vi "all-signals-expressvi-to-TDMS.vi"() -> ()   [LabVIEW 2018]
panel:
  in  "Dateiname":string="test.tdms"
  in  "Dateipfad":path=path "C:/Users/lauri/OneDrive/Dokumente/Uni/HTW/Diplomarbeit/Versuchsstand neu/labview/messungen"
  in  "Stop Measurement (F)":bool caption="Messung stoppen, Counter schreiben (F)"
  in  "Clear Charts":bool
  in  "Messzeit in ms":u32=100 min=10 max=1000 step=10
  out "Bremsmoment":waveform(dbl)(graph)
  out "Strom, Spannung, elektrische Leistung":dynamicdata(graph)
  out "Counter/Messzeit":waveform(dbl)(graph)
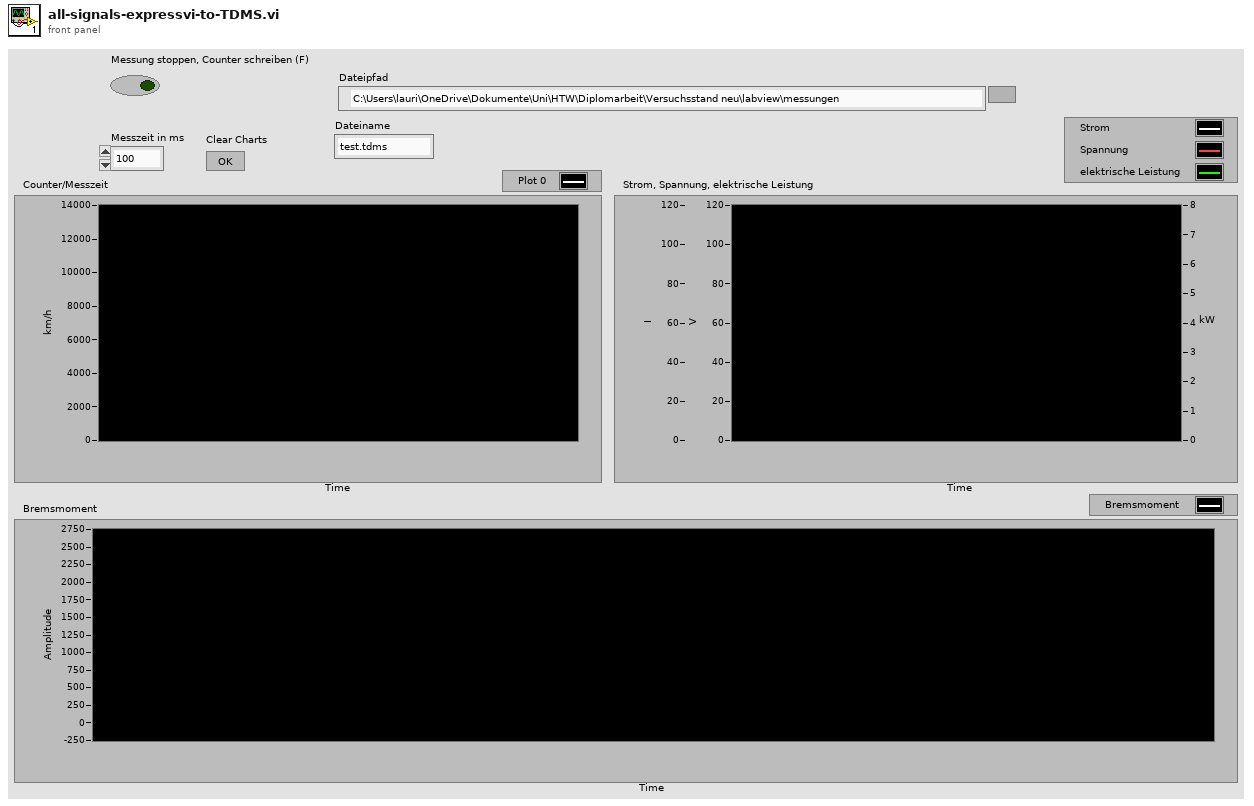
[diagram p1: front panel]
types:
  T1 = enum16{"open", "open or create", "create or replace", "create", "open (read-only)"}
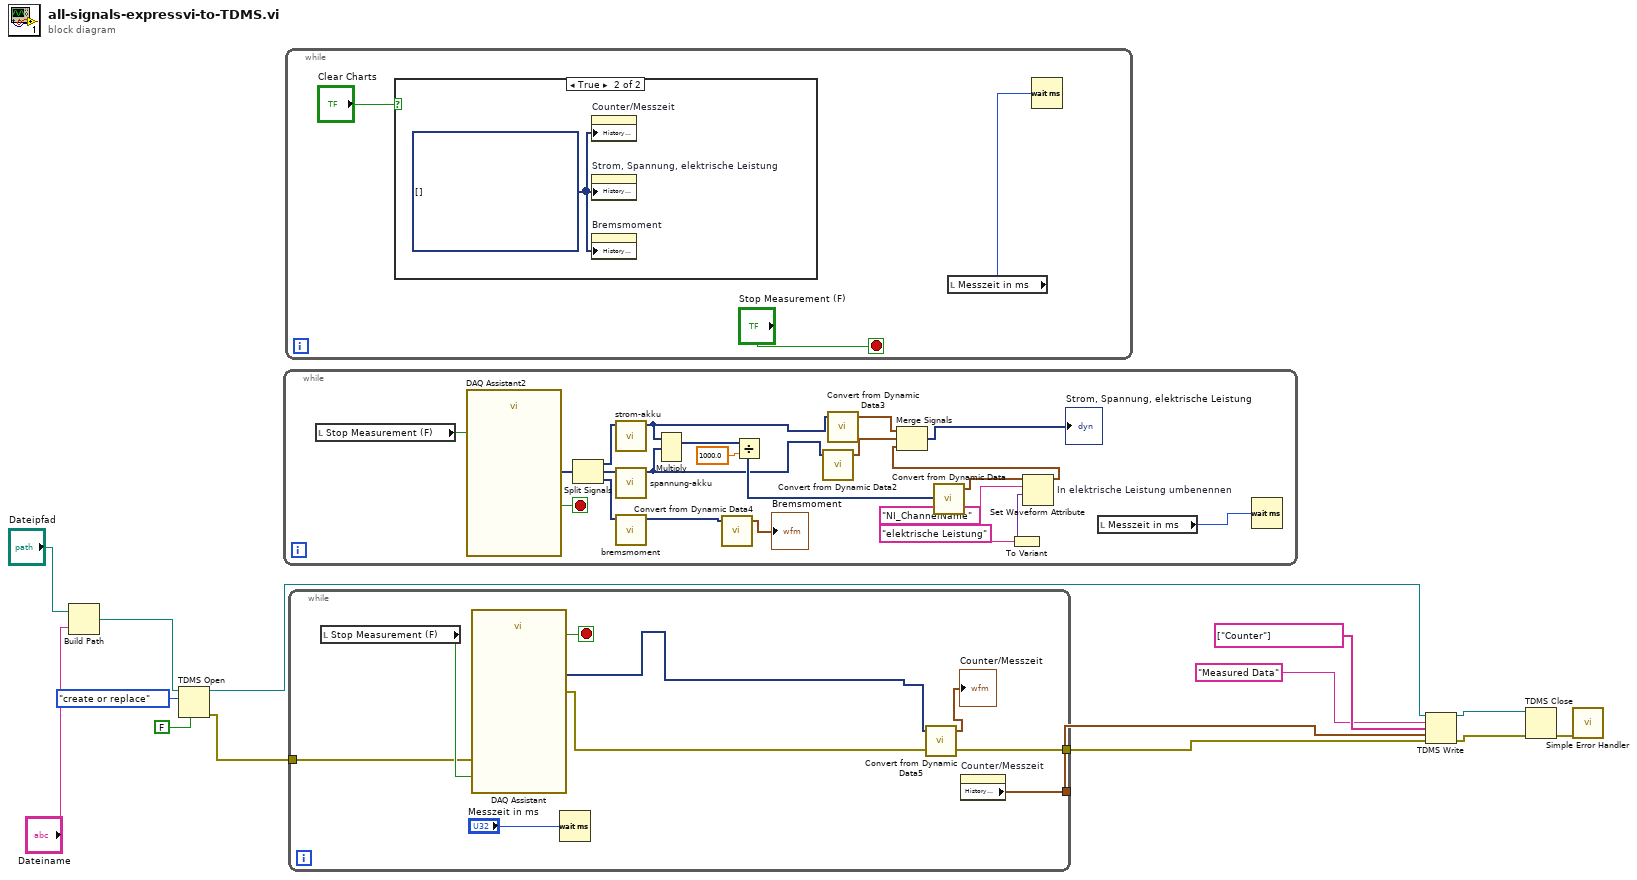
[diagram p0: block diagram]
diagram:
  n1 = Build Path(base path="Dateipfad", name or relative path="Dateiname") -> (appended path=w6:path)
  n2 = TDMS Open(6:FALSE ("disable buffering? (T)"), 10:T1."create or replace" ("operation (0:open)"), 11:w6) -> (0:w11:errorcluster, 3:w8:refnum<k34>)  [unwired: 4 in]
  n3 = while {
    stop <- w32 stop-if-true
    n4 = local read "Stop Measurement (F)"() -> (w29:bool)
    n5 = call "DAQ Assistant2"("stop (F)"=w29) -> ("data"=w33:dynamicdata, "stopped"=w32:bool)  [unwired: 15 in, 2 out]
    n6 = Split Signals(w33) -> (w36:dynamicdata, w35:dynamicdata, w34:dynamicdata)  [unwired: 3 in]
    n7 = call "strom-akku.vi"("Dynamic Data"=w36) -> ("Filtered Signal"=w20:dynamicdata)  [unwired: 10 in]
    n8 = call "spannung-akku.vi"("Dynamic Data in"=w35) -> ("Dynamic Data out"=w22:dynamicdata)  [unwired: 10 in]
    n9 = call "bremsmoment.vi"("Dynamic Data in"=w34) -> ("Dynamic Data out"=w18:dynamicdata)  [unwired: 10 in]
    n10 = Multiply(1:w22, 2:w20) -> (0:w30:dynamicdata)  [unwired: 1 in, 1 out]
    n11 = call "Convert from Dynamic Data4"("Dynamic Data Type"=w18) -> ("Waveform"=→"Bremsmoment":waveform(dbl))  [unwired: 3 in]
    n12 = Divide(x=w30, y=1000.0) -> (x/y=w28:dynamicdata)
    n13 = call "Convert from Dynamic Data2"("Dynamic Data Type"=w22) -> ("Waveform"=w21:waveform(dbl))  [unwired: 3 in]
    n14 = call "Convert from Dynamic Data3"("Dynamic Data Type"=w20) -> ("Waveform"=w19:waveform(dbl))  [unwired: 3 in]
    n15 = call "Convert from Dynamic Data"("Dynamic Data Type"=w28) -> ("Waveform"=w24:waveform(dbl))  [unwired: 3 in]
    n16 = To Variant(anything="elektrische Leistung") -> (Variant=w27:variant)
    n17 = Set Waveform Attribute "In elektrische Leistung umbenennen"(5:w27, 6:"NI_ChannelName" ("name"), 7:w24) -> (3:w23:waveform(dbl))  [unwired: 1 in, 2 out]
    n18 = Merge Signals "Merge Signals"(w19, w21, w23) -> (→"Strom, Spannung, elektrische Leistung":dynamicdata)
    n19 = local read "Messzeit in ms"() -> (w15:u32)
    n20 = Wait (ms)(milliseconds to wait=w15) -> ()  [unwired: 1 out]
  }
  n21 = while {
    stop <- "Stop Measurement (F)" stop-if-true
    n22 = case shown="True" "Clear Charts" {
      frame False {
      }
      frame True {
        w40 = dynamicdata[] [] ("History Data")
        n23 = property on="Counter/Messzeit" class="WFChart (strict)"("History Data"=w40) -> ()  [unwired: 2 in, 2 out]
        n24 = property on="Strom, Spannung, elektrische Leistung" class="WFChart (strict)"("History Data"=w40) -> ()  [unwired: 2 in, 2 out]
        n25 = property on="Bremsmoment" class="WFChart (strict)"("History Data"=w40) -> ()  [unwired: 2 in, 2 out]
      }
    }
    n26 = local read "Messzeit in ms"() -> (w37:u32)
    n27 = Wait (ms)(milliseconds to wait=w37) -> ()  [unwired: 1 out]
  }
  n28 = while {
    tunnel: [w45] -> w14
    tunnel: w11 -> [w44]
    tunnel: [w43] -> w10
    stop <- w48 stop-if-true
    n29 = local read "Stop Measurement (F)"() -> (w47:bool)
    n30 = call "DAQ Assistant"("error in"=w44, "stop (F)"=w47) -> ("data"=w41:dynamicdata, "stopped"=w48:bool, "error out"=w43:errorcluster)  [unwired: 14 in, 1 out]
    n31 = Wait (ms)(milliseconds to wait="Messzeit in ms") -> ()  [unwired: 1 out]
    n32 = call "Convert from Dynamic Data5"("Dynamic Data Type"=w41) -> ("Waveform"=→"Counter/Messzeit":waveform(dbl))  [unwired: 3 in]
    n33 = property on="Counter/Messzeit" class="WFChart (strict)"() -> ("History Data"=w45:waveform(dbl)[])  [unwired: 2 in, 2 out]
  }
  n34 = TDMS Write(0:w8, 5:"Measured Data" ("group name in (Untitled)"), 7:string[] ["Counter"] ("channel name(s) in (Untitled)"), 9:w14, 11:w10) -> (4:w1:refnum<k34>, 15:w2:errorcluster)  [unwired: 1 in, 2 out]
  n35 = TDMS Close(8:w2, 11:w1) -> (0:w3:errorcluster)  [unwired: 1 out]
  n36 = call <vilib>:"Simple Error Handler.vi"("error in (no error)"=w3) -> ()  [unwired: 2 in, 7 out]
